vi "Write Addr.vi"(8 "error in (no error)":errorcluster, 10 "Addr":string, 11 "Pressure Monitor in":refnum<class "Pressure Monitor.lvclass">) -> (0 "error out":errorcluster, 3 "Pressure Monitor out":refnum<class "Pressure Monitor.lvclass">)   [LabVIEW 2022 SP3, in "Pressure Monitor.lvclass"]
uses:
  Pressure Monitor.lvclass
  Pressure Monitor.lvclass/Pressure Monitor.ctl
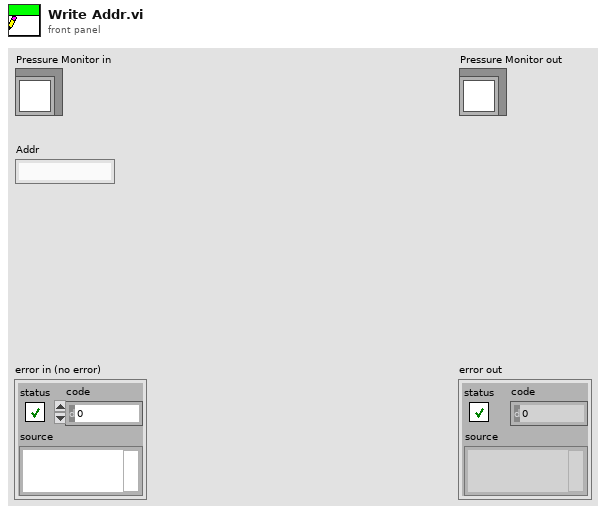
[diagram p1: front panel]
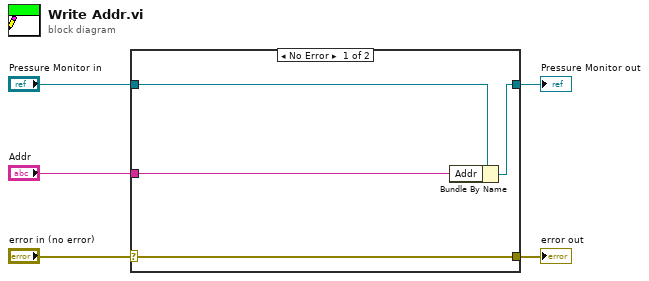
[diagram p0: block diagram]
diagram:
  n1 = case shown="No Error" "error in (no error)" {
    selector: "error in (no error)" -> [w9 w10]
    tunnel: [w9 w10] -> w4
    tunnel: [w7 w11] -> w2
    tunnel: "Pressure Monitor in" -> [w8 w11]
    tunnel: "Addr" -> [w6 _]
    frame No Error {
      n2 = Bundle By Name(cluster=w8, "Addr"=w6) -> (w7:refnum<class "Pressure Monitor.lvclass">)
    }
    frame Error {
    }
  }
  "error out" <- w4
  "Pressure Monitor out" <- w2
